vi "Plot_add_to_buffer.vi"(2 "Plot parameters in":T1, 3 "fast mode":enum16{"normal sweep", "fast sweep"}(ring), 4 "Points":cluster{string, "data":u64, "data":dbl}[](array[cluster])=[{"0:0", "data"=0, "data"=-0.0}], 5 "new_data":dbl[][][](array[numeric]), 6 "sweep_dim":u64[](array[numeric])=[11, 61, 61], 7 "Indexes":i32[](array[numeric])=[8, 21, 0]) -> (0 "Plot parameters out":T1)   [LabVIEW 2013]
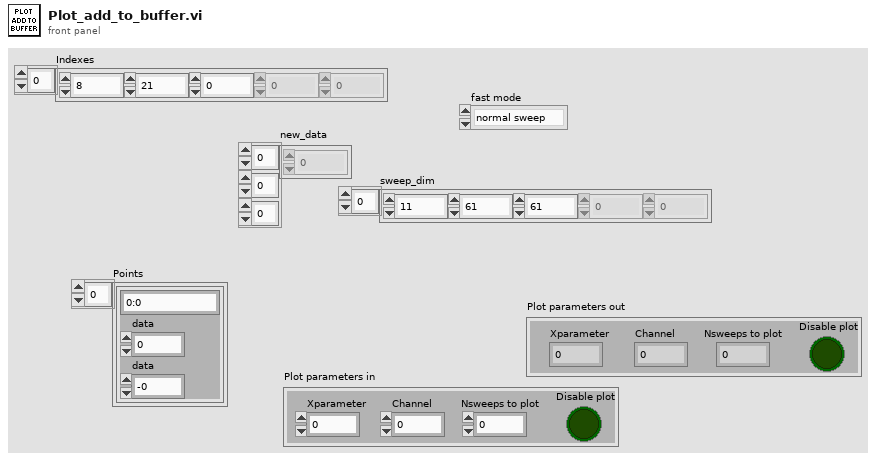
[diagram p1: front panel]
types:
  T1 = cluster{"Disable plot":bool, "Nsweeps to plot":dbl, "Channel":dbl, "Xparameter":dbl, "Readout buffer":dbl[][], "Sweep buffer":dbl[][]}
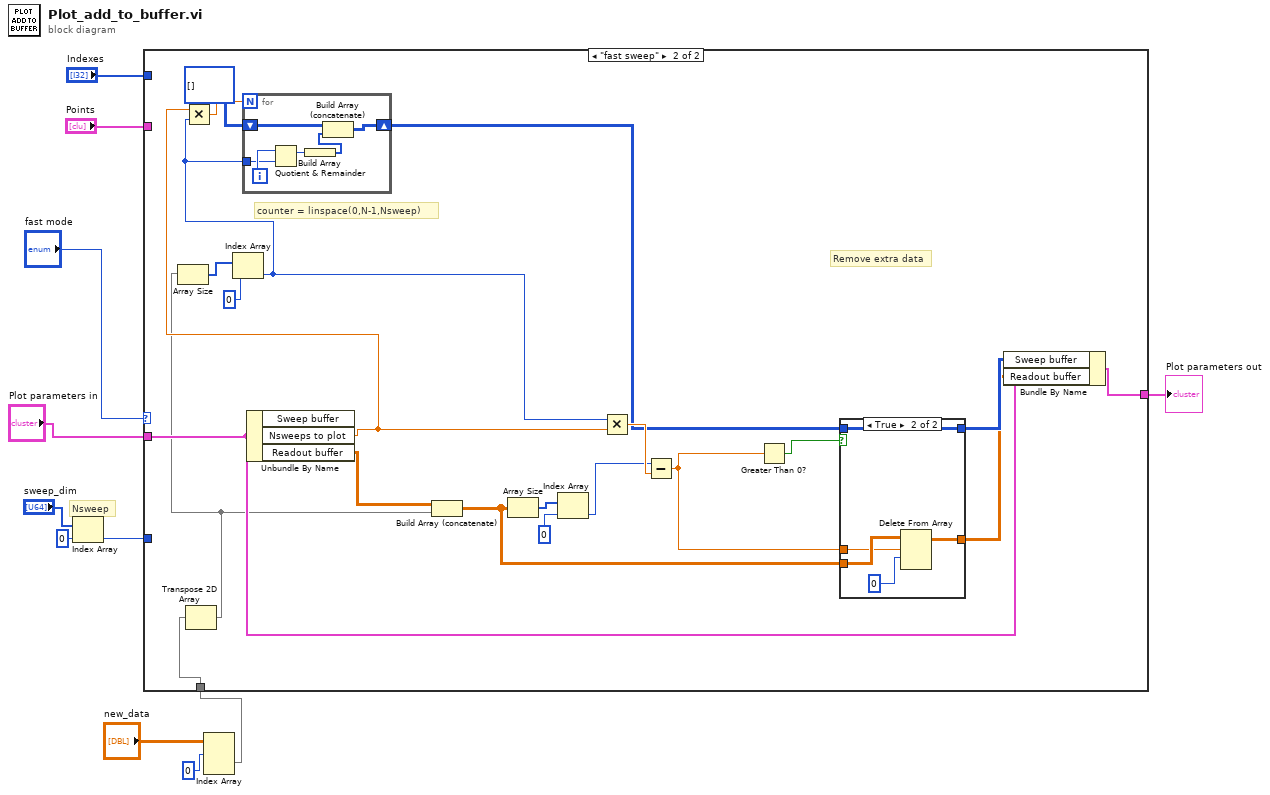
[diagram p0: block diagram]
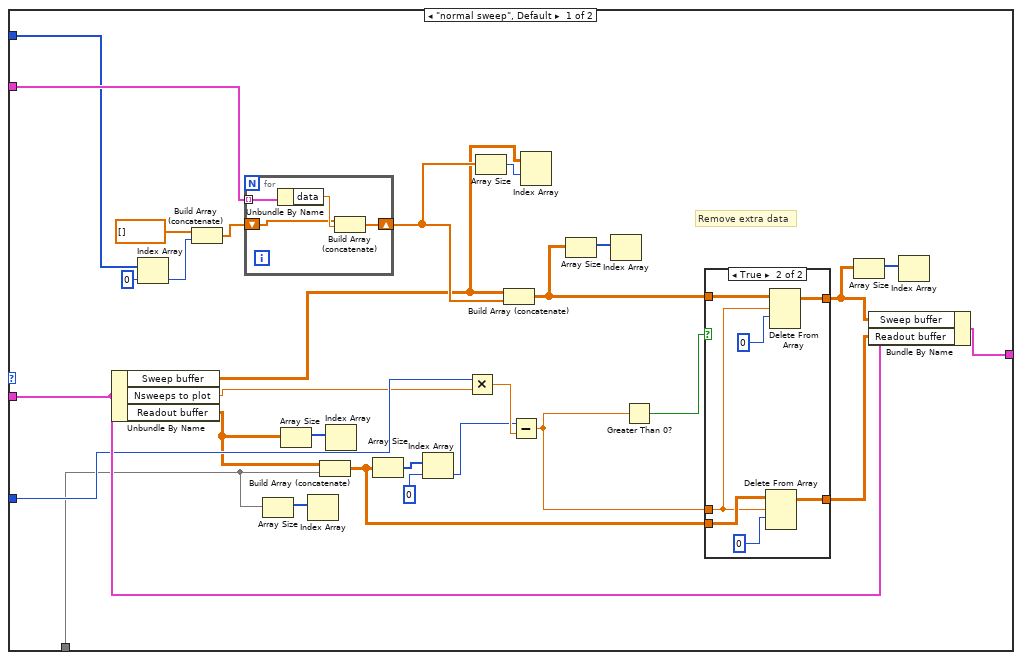
[diagram p2: hidden frame]
diagram:
  # "Nsweep"
  n1 = Index Array(array="sweep_dim", index=0) -> (element=w6:u64)
  n2 = Index Array(array="new_data", index (dim 0)=0 ("disabled index (col)")) -> (element=w2:dbl[][])  [unwired: 2 in]
  n3 = case shown="\"fast sweep\"" "fast mode" {
    tunnel: "Plot parameters in" -> [w28 w68]
    tunnel: [w27 w67] -> w10
    tunnel: w6 -> [w26 _]
    tunnel: w2 -> [w13 w54]
    tunnel: "Points" -> [w24 _]
    tunnel: "Indexes" -> [w23 _]
    frame "normal sweep", Default {
      # "Remove extra data"
      n4 = Unbundle By Name(w28) -> ("Sweep buffer"=w16:dbl[][], "Nsweeps to plot"=w25:dbl, "Readout buffer"=w14:dbl[][])
      n5 = Index Array(array=w23, index=0) -> (element=w29:i32)
      n6 = Build Array (concatenate)(dbl[] [], w29) -> (w30:dbl[])
      n7 = for {
        tunnel: w24 -> [w42] mode=indexing
        shift-right: [w44] -> w22
        shift-left: w30 -> [w41]
        n8 = Unbundle By Name(w42) -> ("data"=w43:dbl)
        n9 = Build Array (concatenate)(w41, w43) -> (w44:dbl[])
      }
      n10 = Array Size(array=w13) -> (size(s)=w12:i32[])
      n11 = Array Size(array=w14) -> (size(s)=w15:i32[])
      n12 = Index Array(array=w12) -> ()  [unwired: 1 in, 1 out]
      n13 = Build Array (concatenate)(w14, w13) -> (w37:dbl[][])
      n14 = Index Array(array=w15) -> ()  [unwired: 1 in, 1 out]
      n15 = Array Size(array=w37) -> (size(s)=w40:i32[])
      n16 = Index Array(array=w40, index=0) -> (element=w35:i32)
      n17 = Multiply(x=w26, y=w25) -> (x*y=w36:dbl)
      n18 = Array Size(array=w22) -> (size(s)=w21:i32)
      n19 = Build Array (concatenate)(w16, w22) -> (w19:dbl[][])
      n20 = Subtract(x=w35, y=w36) -> (x-y=w34:dbl)
      n21 = Index Array(array=w16, index (row)=w21) -> ()  [unwired: 1 in, 1 out]
      n22 = Array Size(array=w19) -> (size(s)=w20:i32[])
      n23 = Index Array(array=w20) -> ()  [unwired: 1 in, 1 out]
      n24 = Greater Than 0?(x=w34) -> (x > 0?=w38:bool)
      n25 = case shown="True" w38 {
        tunnel: w37 -> [w46 w52]
        tunnel: w34 -> [_ w49]
        tunnel: [w46 w51] -> w33
        tunnel: [w45 w48] -> w17
        tunnel: w19 -> [w45 w47]
        frame False {
        }
        frame True {
          n26 = Delete From Array(array=w52, length=w49, index (row)=0) -> (array with subset deleted=w51:dbl[][])  [unwired: 1 in, 1 out]
          n27 = Delete From Array(array=w47, length=w49, index (row)=0) -> (array with subset deleted=w48:dbl[][])  [unwired: 1 in, 1 out]
        }
      }
      n28 = Array Size(array=w17) -> (size(s)=w18:i32[])
      n29 = Bundle By Name(cluster=w28, "Sweep buffer"=w17, "Readout buffer"=w33) -> (w27:T1)
      n30 = Index Array(array=w18) -> ()  [unwired: 1 in, 1 out]
    }
    frame "fast sweep" {
      # "counter = linspace(0,N-1,Nsweep)"
      # "Remove extra data"
      n31 = Transpose 2D Array(2D array=w54) -> (transposed array=w55:dbl[][])
      n32 = Array Size(array=w55) -> (size(s)=w66:i32[])
      n33 = Index Array(array=w66, index=0) -> (element=w56:i32)
      n34 = Unbundle By Name(w68) -> ("Nsweeps to plot"=w61:dbl, "Readout buffer"=w59:dbl[][])  [unwired: 1 out]
      n35 = Multiply(x=w61, y=w56) -> (x*y=w60:dbl)
      n36 = for {
        N: w60 -> [_]
        shift-right: [w79] -> w58
        shift-left: i32[][] [] -> [w80]
        tunnel: w56 -> [w75]
        i -> [w78]
        n37 = Quotient & Remainder(x=w78, y=w75) -> (x-y*floor(x/y)=w76:i32)  [unwired: 1 out]
        n38 = Build Array(w76) -> (w77:i32[])
        n39 = Build Array (concatenate)(w80, w77) -> (w79:i32[][])
      }
      n40 = Build Array (concatenate)(w59, w55) -> (w62:dbl[][])
      n41 = Array Size(array=w62) -> (size(s)=w74:i32[])
      n42 = Index Array(array=w74, index=0) -> (element=w70:i32)
      n43 = Multiply(x=w56, y=w61) -> (x*y=w71:dbl)
      n44 = Subtract(x=w70, y=w71) -> (x-y=w69:dbl)
      n45 = Greater Than 0?(x=w69) -> (x > 0?=w72:bool)
      n46 = case shown="True" w72 {
        tunnel: w62 -> [w82 w86]
        tunnel: w69 -> [_ w84]
        tunnel: [w82 w85] -> w63
        tunnel: [w81 w83] -> w64
        tunnel: w58 -> [w81 w83]
        frame False {
        }
        frame True {
          n47 = Delete From Array(array=w86, length=w84, index (row)=0) -> (array with subset deleted=w85:dbl[][])  [unwired: 1 in, 1 out]
        }
      }
      n48 = Bundle By Name(cluster=w68, "Sweep buffer"=w64, "Readout buffer"=w63) -> (w67:T1)
    }
  }
  "Plot parameters out" <- w10
